vi "Generator.vi"(2 "R":bool, 3 "T ms (500)":u32=500, 4 "ON (F)":bool) -> (1 "Q":bool)   [LabVIEW 2019, in "Counter.lvlib"]
uses:
  Counter.lvlib
  Trigers/Triggers.lvlib
  Timer Delay/Timers.lvlib
  Logik/Logik.lvlib
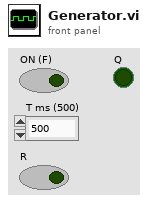
[diagram p1: front panel]
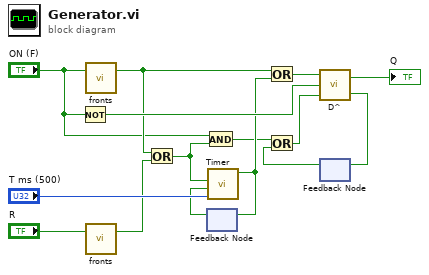
[diagram p0: block diagram]
diagram:
  n1 = Not(x="ON (F)") -> (.not. x?=w12:bool)
  n2 = call "fronts.vi"("in"="ON (F)") -> ("raise"=w8:bool)  [unwired: 1 in, 1 out]
  n3 = call "fronts.vi"("in"="R") -> ("raise"=w7:bool)  [unwired: 1 in, 1 out]
  n4 = Or(x=w8, y=w7) -> (x .or. y?=w3:bool)
  n5 = And(x="ON (F)", y=w3) -> (x .and. y?=w1:bool)
  n6 = feedback #1() -> (w11:bool)  [unwired: 1 in]
  n7 = call "Timer.vi"("ms"="T ms (500)", "Load (F)"=w11, "Reset (F)"=w3) -> ("End"=w10:bool)  [unwired: 6 in, 1 out]
  n8 = feedback-in #1(w10) -> ()
  n9 = Or(x=w8, y=w10) -> (x .or. y?=w6:bool)
  n10 = feedback #2() -> (w5:bool)  [unwired: 1 in]
  n11 = Or(x=w1, y=w5) -> (x .or. y?=w4:bool)
  n12 = call "D^.vi"("D"=w4, "R"=w12, "^"=w6) -> ("~Q"=w15:bool, "Q"=→"Q":bool)
  n13 = feedback-in #2(w15) -> ()
